vi "GetTicksNS.vi"(8 "No Error":errorcluster) -> (0 "error out":errorcluster, 3 "ticks [ns]":u64)   [LabVIEW 2024, in "SDL3.lvlib" / "Timer.lvlib"]
doc: "<B>Summary</B>\nGet the number of nanoseconds since SDL library initialization.\n\n<B>Return Value</B>\nReturns an unsigned 64-bit value representing the number of nanoseconds since the SDL library initialized."
uses:
  Timer.lvlib
  Lib/SDL3-32.dll
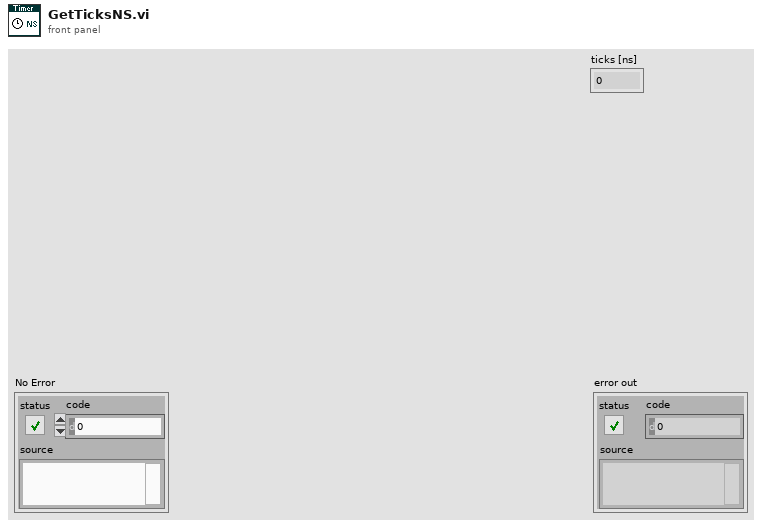
[diagram p1: front panel]
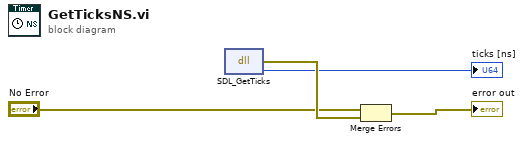
[diagram p0: block diagram]
diagram:
  n1 = dll-call lib="C:/Users/Thomas/Documents/Projects/LV-SDL3/Lib/SDL3-*.*" fn="SDL_GetTicks"() -> (error out=w4:errorcluster, "return type"=→"ticks [ns]":u64)  [unwired: 3 in, 1 out]
  n2 = Merge Errors("No Error", w4) -> (→"error out":errorcluster)
